vi "History_Array_ph.vi"(1 "Current Value":dbl, 2 "Desired Length":i32, 3 "History In":dbl[](array[numeric])) -> (0 "History Out":dbl[](array[numeric]))   [LabVIEW 2011]
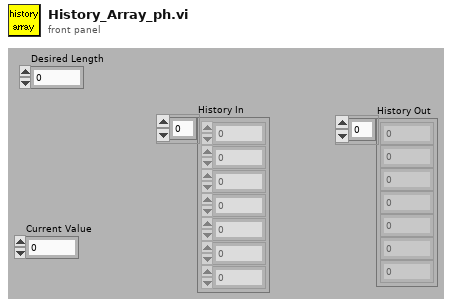
[diagram p1: front panel]
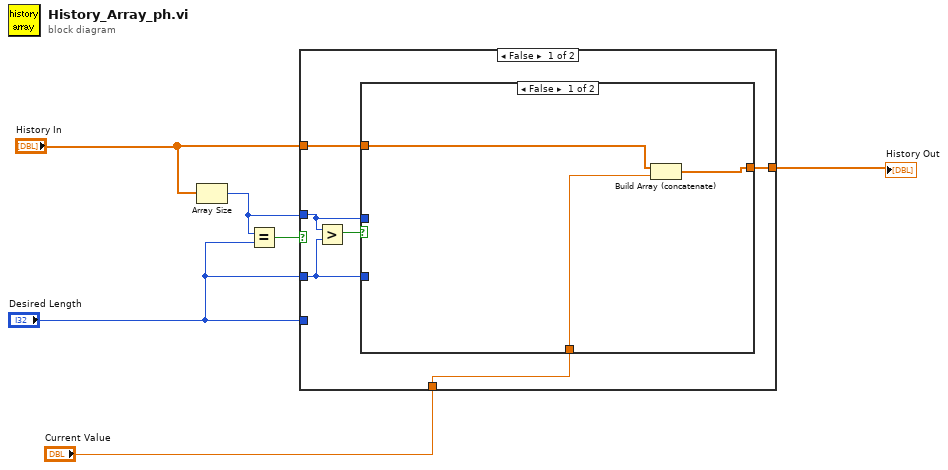
[diagram p0: block diagram]
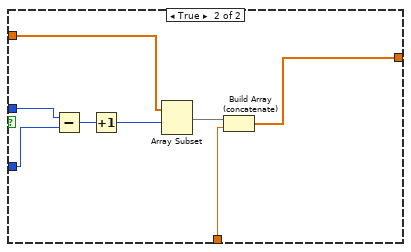
[diagram p2: hidden frame]
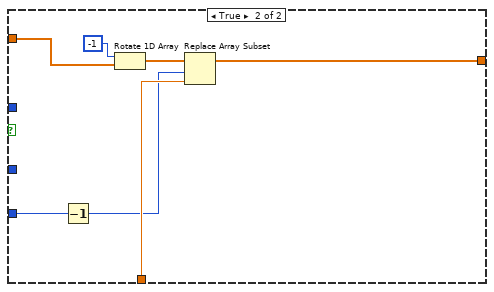
[diagram p3: hidden frame]
diagram:
  n1 = Array Size(array="History In") -> (size(s)=w2:i32)
  n2 = Equal?(x=w2, y="Desired Length") -> (x = y?=w4:bool)
  n3 = case shown="False" w4 {
    tunnel: "History In" -> [w9 w30]
    tunnel: "Current Value" -> [w7 w28]
    tunnel: "Desired Length" -> [_ w26]
    tunnel: [w8 w24] -> w3
    tunnel: w2 -> [w11 _]
    tunnel: "Desired Length" -> [w10 _]
    frame False {
      n4 = Greater?(x=w11, y=w10) -> (0:w12:bool)
      n5 = case shown="False" w12 {
        tunnel: w11 -> [_ w23]
        tunnel: w10 -> [_ w22]
        tunnel: w9 -> [w15 w19]
        tunnel: [w13 w17] -> w8
        tunnel: w7 -> [w14 w16]
        frame False {
          n6 = Build Array (concatenate)(w15, w14) -> (w13:dbl[])
        }
        frame True {
          n7 = Subtract(x=w23, y=w22) -> (x-y=w21:i32)
          n8 = Increment(x=w21) -> (x+1=w20:i32)
          n9 = Array Subset(array=w19, index=w20) -> (w18:dbl[])  [unwired: 1 in]
          n10 = Build Array (concatenate)(w18, w16) -> (w17:dbl[])
        }
      }
    }
    frame True {
      n11 = Decrement(x=w26) -> (x-1=w25:i32)
      n12 = Rotate 1D Array(1:w30, 2:-1 ("n")) -> (0:w27:dbl[])
      n13 = Replace Array Subset(array=w27, new element=w28, index=w25) -> (w24:dbl[])
    }
  }
  "History Out" <- w3
